vi "Multiple Roots Visualization.vi"() -> ()   [LabVIEW 2017, in "Tree API.lvlib" / "Tree.lvclass"]
uses:
  Tree.lvclass
panel:
  out "All Names":string[](array[string])=["Child 3", "Parent 1", "Child 2", "Parent 2", "Child 1"]
  out "All IDs":string[](array[string])=["GDyiH8xC8K2eXxAD", "J1GTkAhb8Y8anQWl", "fRClFkPRThmhJCCu", "h2yLWdqAgvQAAIFp", "mh36Ej5eWly8kXuV"]
  out "Roots Names":string[](array[string])=["Parent 1", "Parent 2"]
  out "Roots IDs":string[](array[string])=["J1GTkAhb8Y8anQWl", "h2yLWdqAgvQAAIFp"]
  in  "Tree 2":string(tree)
  in  "Tree":string(tree)
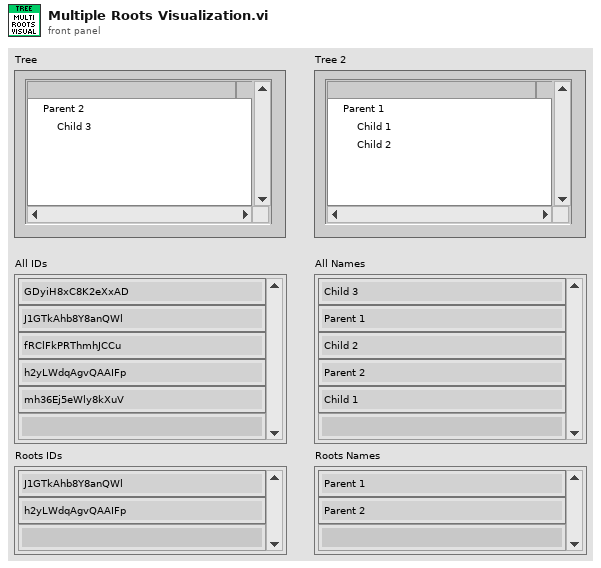
[diagram p1: front panel]
types:
  T1 = cluster{"Left Cell String":string, "Child Text":string[], "Child Tag":string, "Item Indent":i32, "Child Only?":bool, "Glyph Index":i32}[]
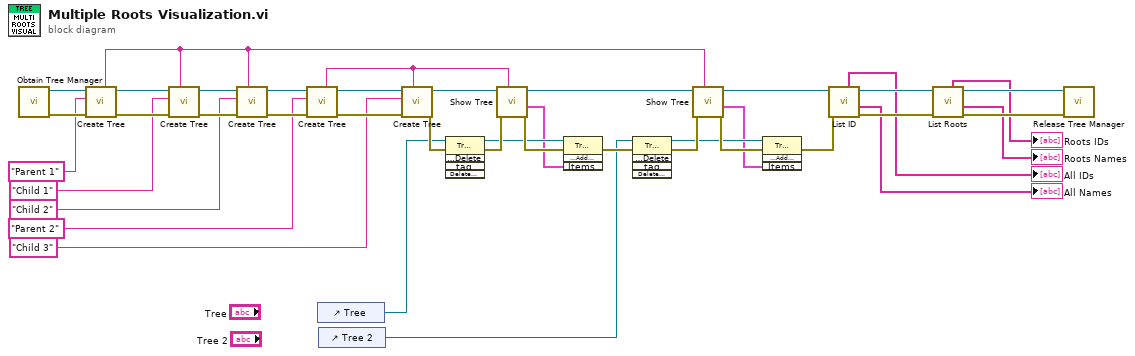
[diagram p0: block diagram]
diagram:
  n1 = call "Obtain Tree Manager.vi"() -> ("Error Out"=w40:errorcluster, "Tree"=w41:refnum<data-value>)  [unwired: 10 in]
  n2 = call "Create Tree.vi"("Error In"=w40, "Name"="Parent 1", "Tree Manager"=w41) -> ("Error Out"=w38:errorcluster, "Tree Manager"=w39:refnum<data-value>, "Unique ID"=w14:string)  [unwired: 6 in]
  n3 = call "Create Tree.vi"("Parent ID (empty)"=w14, "Error In"=w38, "Name"="Child 1", "Tree Manager"=w39) -> ("Error Out"=w36:errorcluster, "Tree Manager"=w37:refnum<data-value>)  [unwired: 5 in, 1 out]
  n4 = call "Create Tree.vi"("Parent ID (empty)"=w14, "Error In"=w36, "Name"="Child 2", "Tree Manager"=w37) -> ("Error Out"=w34:errorcluster, "Tree Manager"=w35:refnum<data-value>)  [unwired: 5 in, 1 out]
  n5 = call "Create Tree.vi"("Error In"=w34, "Name"="Parent 2", "Tree Manager"=w35) -> ("Error Out"=w32:errorcluster, "Tree Manager"=w33:refnum<data-value>, "Unique ID"=w19:string)  [unwired: 6 in]
  n6 = control-ref of="Tree"() -> (w11:refnum<vi>)
  n7 = control-ref of="Tree 2"() -> (w6:refnum<vi>)
  n8 = call "Create Tree.vi"("Parent ID (empty)"=w19, "Error In"=w32, "Name"="Child 3", "Tree Manager"=w33) -> ("Error Out"=w13:errorcluster, "Tree Manager"=w31:refnum<data-value>)  [unwired: 5 in, 1 out]
  n9 = invoke class="Tree (strict)" method="Edit Tree Items.Delete"(reference=w11, error in=w13) -> (reference out=w9:refnum<vi>, error out=w12:errorcluster)  [unwired: 3 in, 3 out]
  n10 = call "Show Tree.vi"("Root ID"=w19, "Error In"=w12, "Tree"=w31) -> ("Error Out"=w10:errorcluster, "Items Out"=w2:T1, "Tree"=w24:refnum<data-value>)  [unwired: 6 in]
  n11 = invoke class="Tree (strict)" method="Edit Tree Items.Add Multiple Items to End"(reference=w9, error in=w10, "Items"=w2) -> (error out=w8:errorcluster)  [unwired: 1 in, 3 out]
  n12 = invoke class="Tree (strict)" method="Edit Tree Items.Delete"(reference=w6, error in=w8) -> (reference out=w4:refnum<vi>, error out=w7:errorcluster)  [unwired: 3 in, 3 out]
  n13 = call "Show Tree.vi"("Root ID"=w14, "Error In"=w7, "Tree"=w24) -> ("Error Out"=w5:errorcluster, "Items Out"=w1:T1, "Tree"=w23:refnum<data-value>)  [unwired: 6 in]
  n14 = invoke class="Tree (strict)" method="Edit Tree Items.Add Multiple Items to End"(reference=w4, error in=w5, "Items"=w1) -> (error out=w3:errorcluster)  [unwired: 1 in, 3 out]
  n15 = call "List ID.vi"("Error In"=w3, "Tree Manager"=w23) -> ("Error Out"=w21:errorcluster, "Child Names"=→"All Names":string[], "Tree Manager"=w22:refnum<data-value>, "Child IDs"=→"All IDs":string[])  [unwired: 6 in]
  n16 = call "List Roots.vi"("Error In"=w21, "Tree"=w22) -> ("Error Out"=w26:errorcluster, "Roots Names"=→"Roots Names":string[], "Tree"=w25:refnum<data-value>, "Roots IDs"=→"Roots IDs":string[])  [unwired: 6 in]
  n17 = call "Release Tree Manager.vi"("Error In"=w26, "Tree"=w25) -> ()  [unwired: 9 in, 1 out]
